vi "Read Sub Nodes.vi"(8 "error in (no error)":errorcluster, 11 "Composite Tree Data in":refnum<class "Composite Tree Data.lvclass">) -> (0 "error out":errorcluster, 2 "Sub Nodes":refnum<class "Tree Data.lvclass">[](array[class]), 3 "Composite Tree Data out":refnum<class "Composite Tree Data.lvclass">)   [LabVIEW 2019, in "Composite Tree Data.lvclass"]
uses:
  Composite Tree Data.lvclass
  Tree Data/Tree Data.lvclass
  Composite Tree Data.lvclass/Composite Tree Data.ctl
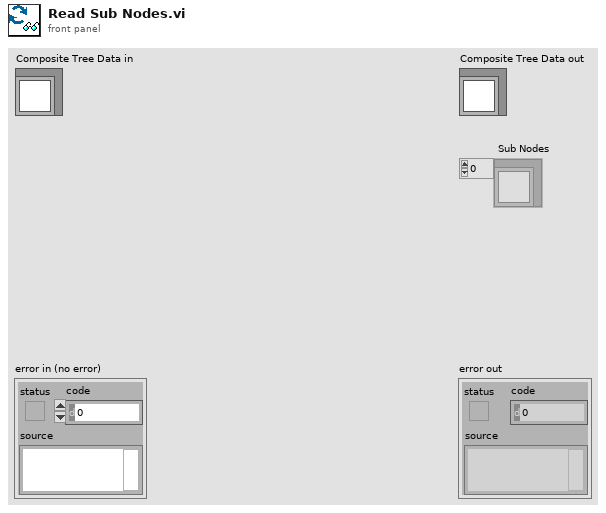
[diagram p1: front panel]
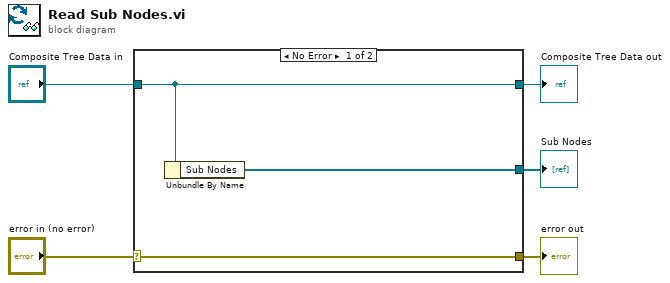
[diagram p0: block diagram]
diagram:
  n1 = case shown="No Error" "error in (no error)" {
    selector: "error in (no error)" -> [w8 w9]
    tunnel: [w8 w9] -> w4
    tunnel: [w7 w10] -> w2
    tunnel: "Composite Tree Data in" -> [w7 w10]
    tunnel: [w6 _] -> w1
    frame No Error {
      n2 = Unbundle By Name(w7) -> ("Sub Nodes"=w6:refnum<class "Tree Data.lvclass">[])
    }
    frame Error {
    }
  }
  "error out" <- w4
  "Composite Tree Data out" <- w2
  "Sub Nodes" <- w1
